vi "Calibration_Save_file.vi"(7 "Current":dbl, 8 "error in (no error)":errorcluster, 10 "Range - Shunts":T1, 11 "DEV SN":u64) -> (0 "error out":errorcluster)   [LabVIEW 2017]
uses:
  Range_Shunt_selector.ctl
  <vilib>/Utility/config.llb/Write Key (Double).vi
  <vilib>/Utility/config.llb/NI_LVConfig.lvlib
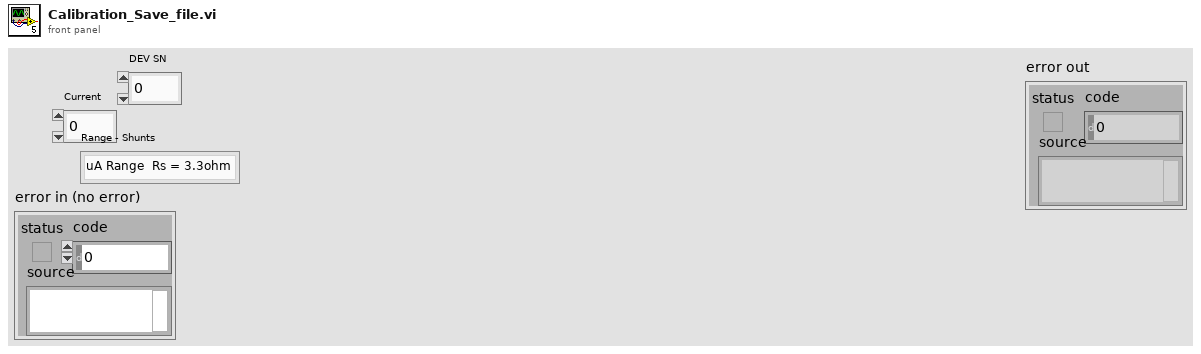
[diagram p1: front panel]
types:
  T1 = typedef "Range_Shunt_selector.ctl" = enum16{"uA Range  Rs = 3.3ohm", "mA Range Rs = 3.3ohm", "mA Range Rs = 1ohm", "mA Range Rs = 1ohm - X2"}
  T2 = typedef "NI_LVConfig.lvlib/Config Data RefNum.ctl" = refnum<k1>
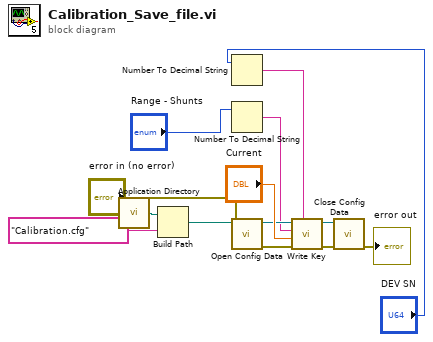
[diagram p0: block diagram]
diagram:
  n1 = call <vilib>:"Application Directory.vi"() -> ("Application Directory"=w12:path)
  n2 = Build Path(base path=w12, name or relative path="Calibration.cfg") -> (appended path=w14:path)
  n3 = Number To Decimal String(number="DEV SN") -> (decimal integer string=w6:string)  [unwired: 1 in]
  n4 = Number To Decimal String(number="Range - Shunts") -> (decimal integer string=w4:string)  [unwired: 1 in]
  n5 = call <vilib>:"Open Config Data.vi"("error in (no error)"="error in (no error)", "configuration file path"=w14) -> ("error out"=w10:errorcluster, "refnum"=w9:T2)  [unwired: 7 in, 1 out]
  n6 = call-poly <vilib>:"Write Key.vi"("section"=w6, "error in (no error)"=w10, "value"="Current", "key"=w4, "refnum"=w9) -> ("error out"=w7:errorcluster, "refnum out"=w8:T2)  [unwired: 4 in, 1 out]
  n7 = call <vilib>:"Close Config Data.vi"("error in (no error)"=w7, "refnum"=w8) -> ("error out"=→"error out":errorcluster)  [unwired: 8 in, 1 out]
